vi "Command Template.vi"(1 "Line":string) -> (0 "Done":bool)   [LabVIEW 2016]
panel:
  in  "Parameters":i32[](array[numeric])=[1]
  in  "Subcommands":string[](array[string])=["test"]
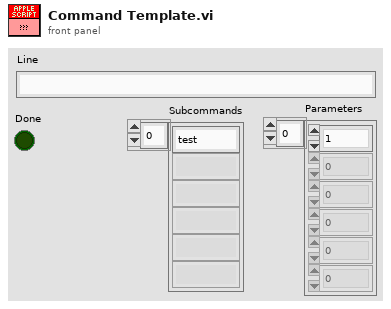
[diagram p1: front panel]
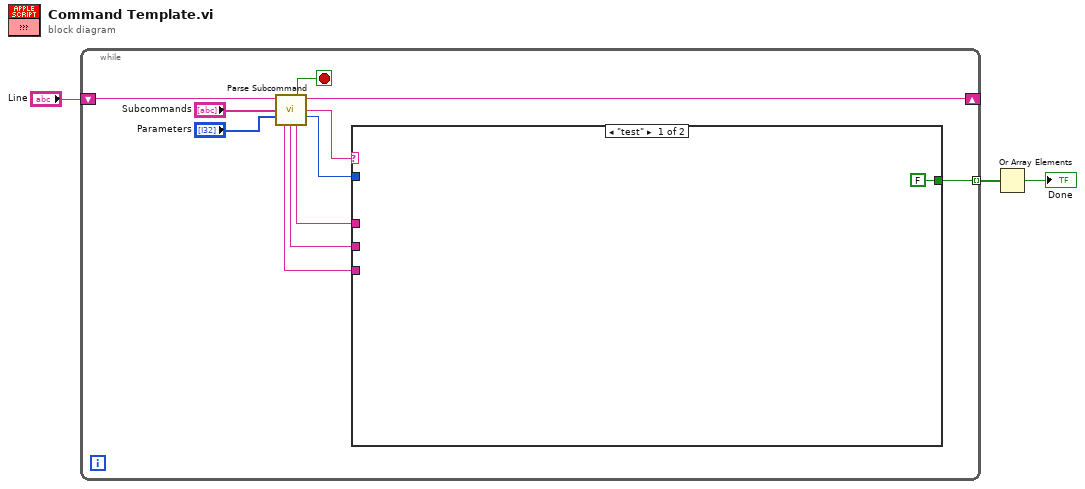
[diagram p0: block diagram]
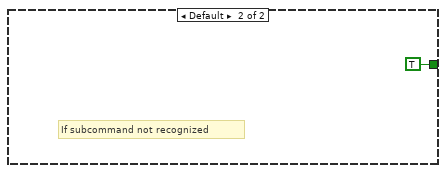
[diagram p2: hidden frame]
diagram:
  n1 = while {
    shift-right: [w11] -> _
    shift-left: "Line" -> [w14]
    tunnel: [w4] -> w2 mode=indexing
    stop <- w10 stop-if-true
    n2 = call "Parse Subcommand.vi"("Text In"=w14, "Subcommands"="Subcommands", "Parameters"="Parameters") -> ("Done"=w10:bool, "Text Out"=w11:string, "Subcommand"=w9:string, "# of Parameters"=w8:i32, "Parameter 3"=w5:string, "Parameter 2"=w6:string, "Parameter 1"=w7:string)  [unwired: 6 in]
    n3 = case shown="\"test\"" w9 {
      tunnel: w8 -> [_ _]
      tunnel: w7 -> [_ _]
      tunnel: w6 -> [_ _]
      tunnel: w5 -> [_ _]
      tunnel: [FALSE TRUE] -> w4
      frame "test" {
      }
      frame Default {
        # "If subcommand not recognized"
      }
    }
  }
  n4 = Or Array Elements(Boolean array=w2) -> (logical OR=→"Done":bool)
